vi "SMBUS Block Read.vi"(4 "WithPEC":u8, 5 "pReadCount":i32, 6 "pReadData":u8, 7 "CommandCode":u8, 9 "SlaveAddr":i16, 10 "IICIndex":i32, 11 "DevHandle":i32) -> (1 "function return":i32, 2 "pReadCount out":i32, 3 "pReadData out":u8)   [LabVIEW 2010, in "usb2iic.lvlib"]
doc: "int WINAPI SMBUS_BlockRead(int DevHandle,int IICIndex,short SlaveAddr,unsigned char CommandCode, unsigned char *pReadData,int *pReadCount,unsigned char WithPEC);"
uses:
  usb2iic.lvlib
  USB2XXX.dll
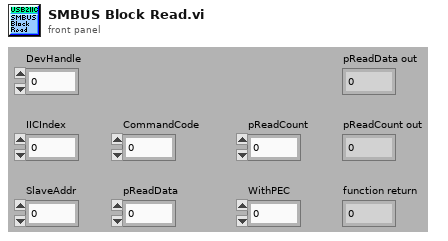
[diagram p1: front panel]
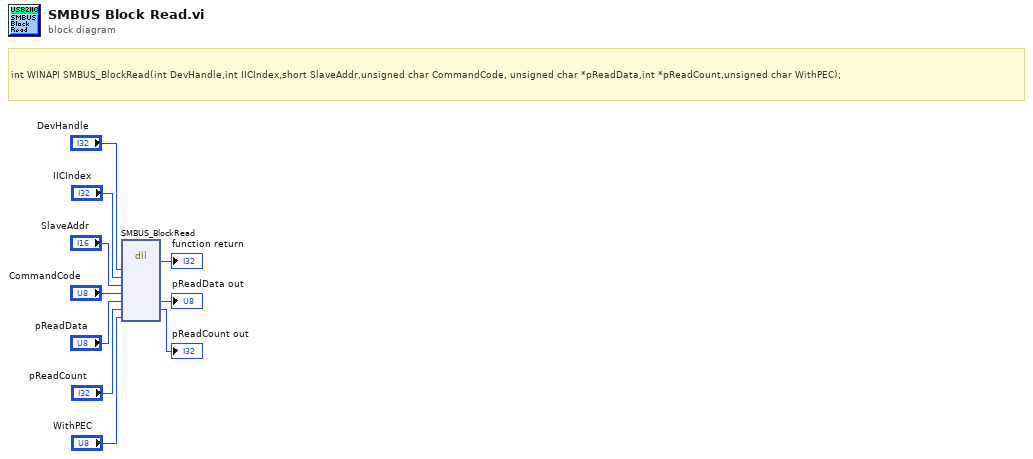
[diagram p0: block diagram]
diagram:
  # "int WINAPI SMBUS_BlockRead(int DevHandle,int IICIndex,short SlaveAddr,unsigned char CommandCode, unsigned char *pReadData,int *pReadCount,unsigned char WithPEC);"
  n1 = dll-call lib="G:/OtherWork/USB2XXX_Example/trunk/Labview/PublicFiles/usb2iic/USB2XXX.*" fn="SMBUS_BlockRead"("DevHandle"="DevHandle", "IICIndex"="IICIndex", "SlaveAddr"="SlaveAddr", "CommandCode"="CommandCode", "pReadData"="pReadData", "pReadCount"="pReadCount", "WithPEC"="WithPEC") -> (→"function return":i32, "pReadData"=→"pReadData out":u8, "pReadCount"=→"pReadCount out":i32)  [unwired: 8 in, 2 out]
